vi "Index to TDMS.Group Name.vi"(8 "error in (no error)":errorcluster, 11 "Append Index":i32) -> (0 "error out":errorcluster, 3 "group name in (Untitled)":string)   [LabVIEW 2016, in "Tranconductance SM.lvclass"]
uses:
  Tranconductance SM.lvclass
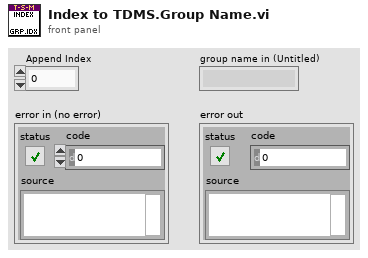
[diagram p1: front panel]
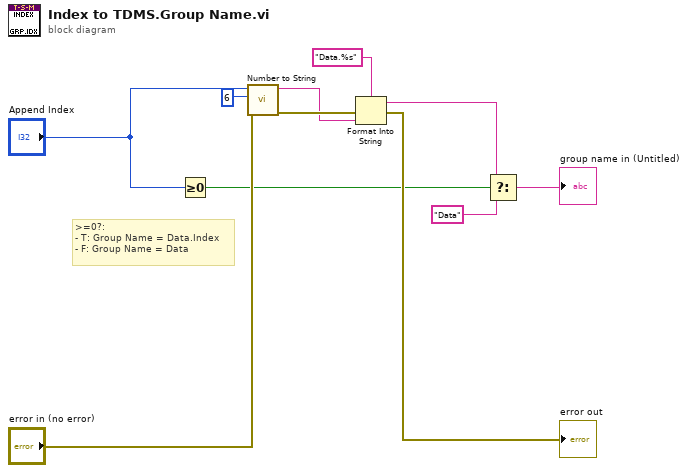
[diagram p0: block diagram]
diagram:
  # ">=0?:\n- T: Group Name = Data.Index\n- F: Group Name = Data"
  n1 = Greater Or Equal To 0?(x="Append Index") -> (x >= 0?=w1:bool)
  n2 = call <userlib>:"Number to String.vi"("error in (no error)"="error in (no error)", "desired minimum string length"=6, "Number"="Append Index") -> ("error out"=w11:errorcluster, "String"=w10:string)  [unwired: 7 in]
  n3 = Format Into String(format string="Data.%s", error in=w11, w10) -> (resulting string=w5:string, error out=→"error out":errorcluster)  [unwired: 1 in]
  n4 = Select(t=w5, s=w1, f="Data" ("group name in (Untitled)")) -> (s? t:f=→"group name in (Untitled)":string)
